vi "Change Tag Data Type.vi"(6 "Variant":variant, 8 "error in":errorcluster, 9 "old values":string[][](array[string]), 10 "object ref in":T2, 11 "Cluster":T3) -> (0 "error out":errorcluster)   [LabVIEW 2013, in "Shared Memory Editor Node.lvclass"]
uses:
  Shared Memory Editor Node.lvclass
  <vilib>/NI/DCAF/Tag Editor Core/Table API/Table Manager/Cell Change.ctl
  <vilib>/NI/DCAF/Tag Editor Core/Table API/Table Manager/object ref.ctl
  <vilib>/NI/DCAF/Tag Editor Core/Configuration Editor/Classes/Engine Parent/Engine Parent Editor Node.lvclass
  <vilib>/NI/DCAF/Tag Editor Core/Configuration Editor/Classes/Module editor node/module editor node.lvclass
  <vilib>/NI/Tag Bus/tag/Data Type.ctl
  module/configuration/Shared Memory Configuration.lvclass
  module/configuration/Shared Memory Configuration.lvclass/Shared Memory Configuration.ctl
  <vilib>/NI/Tag Bus/tag/tag descriptor.lvclass/tag descriptor.ctl
  <vilib>/NI/DCAF/Tag Editor Core/Table API/Table Manager.lvlib
  <vilib>/NI/Tag Bus/tag/tag descriptor.lvclass
  <vilib>/NI/DCAF/Tag Editor Core/Table API/Table Manager/Table Manager.lvclass
panel:
  in  "data type":T1
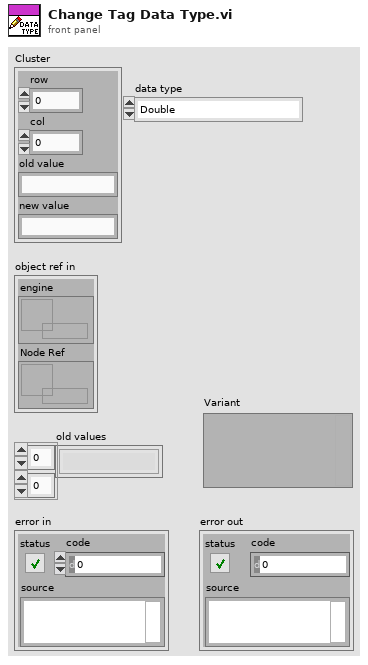
[diagram p1: front panel]
types:
  T1 = typedef "tag bus.lvlib/tag descriptor.lvclass/Data Type.ctl" = enum16{"Double", "Single", "I64", "I32", "I16", "I8", "U64", "U32", "U16", "U8", "Boolean", "String", "Array of Double", "Array of Single", "Array of I64", "Array of I32", "Array of I16", "Array of I8", "Array of U64", "Array of U32", "Array of U16", "Array of U8", "Array of Boolean", "Array of String"}
  T2 = typedef "Table Manager.lvlib/Table Manager.lvclass/object ref.ctl" = cluster{"engine":refnum<data-value>, "Node Ref":refnum<data-value>}
  T3 = typedef "Table Manager.lvlib/Cell Change.ctl" = cluster{"row":i32, "col":i32, "old value":string, "new value":string}
  T4 = typedef "Shared Memory Configuration.lvclass/line configuration.ctl" = cluster{"name":string, "data type":T1, "channel":refnum<class "TBM channel.lvclass">}
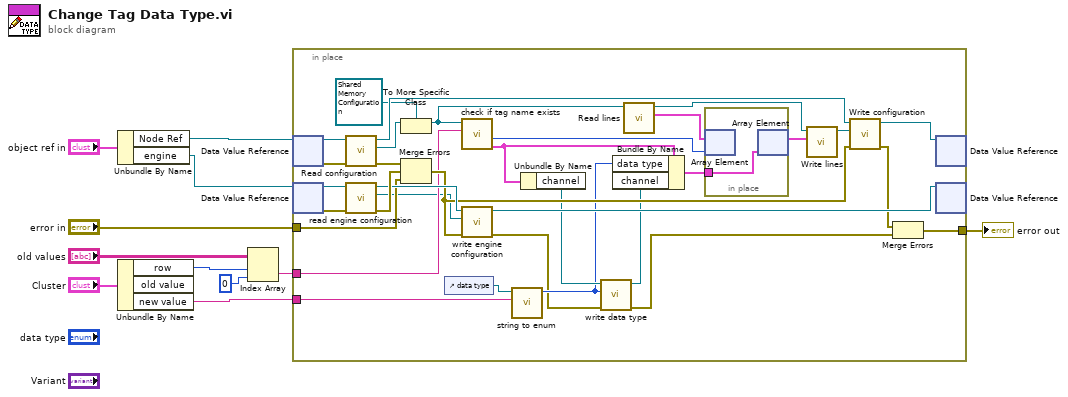
[diagram p0: block diagram]
diagram:
  n1 = Unbundle By Name("object ref in") -> ("Node Ref"=w7:refnum<data-value>, "engine"=w6:refnum<data-value>)
  n2 = Unbundle By Name("Cluster") -> ("row"=w3:i32, "new value"=w5:string)  [unwired: 1 out]
  n3 = Index Array(array="old values", index (row)=w3, index (col)=0 ("disabled index (col)")) -> (element=w1:string)
  n4 = in-place {
    in-place-border: [w37] -> w11
    in-place-border: "error in" -> [w29]
    in-place-border: w1 -> [w23]
    in-place-border: w5 -> [w19]
    n5 = in-place-dvr #1(w7) -> (w34:refnum<class "module editor node.lvclass">, w36:errorcluster)
    n6 = in-place-dvr #2(w6) -> (w43:refnum<class "Engine Parent Editor Node.lvclass">, w44:errorcluster)
    n7 = call-dynamic "Read configuration.vi"("error in"=w36, "NISE_CEF_serializable node in"=w34) -> ("error out"=w35:errorcluster, "configuration"=w32:refnum<class "NISE_CEF_serializable configuration.lvclass">, "NISE_CEF_serializable node out"=w33:refnum<class "module editor node.lvclass">)  [unwired: 7 in]
    n8 = call <vilib>:"read engine configuration.vi"("error in"=w44, "Engine Parent Editor Node in"=w43) -> ("error out"=w40:errorcluster, "engine configuration"=w20:refnum<class "engine configuration.lvclass">, "Engine Parent Editor Node out"=w39:refnum<class "Engine Parent Editor Node.lvclass">)  [unwired: 7 in]
    n9 = To More Specific Class(target class=refnum<class "Shared Memory Configuration.lvclass"> refnum ("tag select module configuration"), reference=w32) -> (specific class reference=w28:refnum<class "Shared Memory Configuration.lvclass">)  [unwired: 1 in, 1 out]
    n10 = Merge Errors(w35, w40, w29) -> (w31:errorcluster)
    n11 = control-ref of="data type"() -> (w18:refnum<vi>)
    n12 = call "check if tag name exists.vi"("name to locate"=w23, "shared memory module configuration in"=w28) -> ("tag config"=w17:T4, "index"=w24:i32)  [unwired: 6 in, 2 out]
    n13 = call <vilib>:"write engine configuration.vi"("error in"=w31, "engine configuration"=w20, "Engine Parent Editor Node in"=w39) -> ("error out"=w13:errorcluster, "Engine Parent Editor Node out"=w42:refnum<class "Engine Parent Editor Node.lvclass">)  [unwired: 7 in]
    n14 = call <vilib>:"string to enum.vi"("String"=w19, "Enum"=w18) -> ("Value"=w15:i32)  [unwired: 8 in, 1 out]
    n15 = Unbundle By Name(w17) -> ("channel"=w16:refnum<class "TBM channel.lvclass">)
    n16 = call <vilib>:"write data type.vi"("error in"=w13, "data type"=w15, "system tag in"=w16) -> ("error out"=w12:errorcluster, "system tag out"=w14:refnum<class "TBM channel.lvclass">)  [unwired: 7 in]
    n17 = Bundle By Name(cluster=w17, "data type"=w15, "channel"=w14) -> (w22:T4)
    n18 = call "Read lines.vi"("shared memory module configuration"=w28) -> ("lines"=w27:T4[], "shared memory module configuration out"=w25:refnum<class "Shared Memory Configuration.lvclass">)  [unwired: 8 in, 1 out]
    n19 = in-place {
      in-place-border: w22 -> [w45]
      n20 = in-place-array #3(w27, w24) -> ()  [unwired: 1 out]
      n21 = in-place-array #3(w45) -> (w26:T4[])  [unwired: 1 out]
    }
    n22 = call "Write lines.vi"("lines"=w26, "shared memory module configuration"=w25) -> ("shared memory module configuration out"=w21:refnum<class "Shared Memory Configuration.lvclass">)  [unwired: 8 in, 1 out]
    n23 = call-dynamic "Write configuration.vi"("error in"=w31, "configuration"=w21, "NISE_CEF_serializable node in"=w33) -> ("error out"=w38:errorcluster, "NISE_CEF_serializable node out"=w41:refnum<class "module editor node.lvclass">)  [unwired: 7 in]
    n24 = Merge Errors(w38, w12) -> (w37:errorcluster)
    n25 = in-place-dvr #1(w41) -> ()  [unwired: 2 out]
    n26 = in-place-dvr #2(w42) -> ()  [unwired: 2 out]
  }
  "error out" <- w11
